vi "RPi HMI Com.vi"(0 "Pump Data":T6={"Voltages"=[0.0, 0.05908203125, 0.06982421875, 0.05908203125, 0.06982421875, 0.0859375], "PumpCurrent"=[0.0015967955457961394, 0.0015950073791676203, 0.0015981739242389562, 0.0015920643549248493, 0.001590499709124895, 0.0015808510600251774], "Speed"=[0.0, 0.0, 0.0, 0.0, 0.0, 0.0], "ControllerCurrent"=[0.0, 0.0, 0.0, 0.0, 0.0, 0.0], "Pressure"=[0.0, 0.0, 0.0, 0.0, 0.0, 0.0], "Flow"=[0.0, 0.0, 0.0, 0.0, 0.0, 0.0], "Elapsed Time (Display)"=[4074.9003000000002, 4074.9003000000002, 4074.9003000000002, 4074.9003000000002, 4074.9003000000002, 4074.9003000000002], "Avg Pressure"=0.0, "Avg Speed"=0.0, "Elapsed Time"=[4074.9003000000002, 4074.9003000000002, 4074.9003000000002, 4074.9003000000002, 4074.9003000000002, 4074.9003000000002]} {"Elapsed Time" format="%<%H:%M:%S>t"; "Elapsed Time (Display)" format="%<%H:%M:%S>t"; "Speed" format="%#_4f"; "ControllerCurrent" format="%#.1g"; "Pressure" format="%#.0f"; "Flow" format="%#.0f"; "PumpCurrent" format="%#.1g"; "Voltages" format="%#.0f"}, 1 "Tank Data":T12 {"PS Actual (V):" format="%.2f"; "Temp1" format="%#_2g"; "Temp2" format="%#_2g"}, 2 "Power Relays":T11, 3 "Pump CMDs":dbl[](array[numeric]), 4 "App Config":T1={"Location"="", "Profiles Path"=path "", "Current Profile"="", "CA Number"="", "Cycles Completed"=0, "Controller Type:"=enum."Kuhnke", "Stagger Time (ms)"=0, "Tank 1 Fuel"="", "Tank 2 Fuel"="", "Serial Numbers"={"Position 1 SN"="", "Position 2 SN"="", "Poaition 3 SN"="", "Position 4 SN"="", "Position 5 SN"="", "Position 6 SN"=""}, "Pumps Present"={"Pump 1"=FALSE, "Pump 2"=FALSE, "Pump 3"=FALSE, "Pump 4"=FALSE, "Pump 5"=FALSE, "Pump 6"=FALSE}, "VoltCtrlRef"="", "VoltageSelect"=FALSE, "Watlow Present"=FALSE, "Temp 1"=0.0, "Temp 2"=0.0, "V_Run PI?"=FALSE, "Voltage Limits"={"V_Step"=1e-05, "V_CmdMax"=0.0, "V_CmdMin"=0.0}, "Voltage Far PI"={"V_FarSlew"=10.0, "V_FarKp"=0.0, "V_FarKi"=0.0}, "Voltage Mid PI"={"V_MidSlew"=10.0, "V_MidKp"=0.0, "V_MidKi"=0.0}, "Voltage Close PI"={"V_CloseSlew"=10.0, "V_CloseKp"=0.0, "V_CloseKi"=0.0}, "Voltage Scale"={"V_FFm"=0.0, "V_FFb"=0.0}, "Voltage Cutoffs"={"V_MidCutoff"=0.0, "V_CloseCutoff"=0.0}, "Pressure Scale"={"Pres_FFm"=1e-05, "Pres_FFb"=0.0}, "Temp Format"=0, "Temp Tolerance"=0.0, "Target Voltage"=0.0, "Target Pressure"=0.0, "Data Log Init"={"Data Path"=path "", "Data Log Rate (S/s)"=0, "AKLH Rate (Hours/S)"=0.0, "Sync Time Offset (min)"=0, "IP Last 3"=0, "WebDAV IP"=""}, "Email Handler IP"="", "ADC Check"=FALSE, "3 Pump Tank"=FALSE, "Cycle Threshold:"=3.0, "Cycle Pts to Avg:"=3, "Anomaly Threshold:"=3.0, "Normal Steps:"=3, "Step Threshold:"=3.0, "Network Drive IP"="", "Network Drive Password"="", "Bank 1 Offset"=0.0, "Bank 2 Offset"=0.0} {"Bank 2 Offset" min=0.0 max=999999.0 step=1.0; "Bank 1 Offset" min=0.0 max=999999.0 step=1.0; "Step Threshold:" min=0.0 max=999999.0 step=1.0; "Normal Steps:" max=999999 step=1; "Anomaly Threshold:" min=0.0 max=999999.0 step=1.0; "Cycle Pts to Avg:" max=999999 step=1; "Cycle Threshold:" min=0.0 max=999999.0 step=1.0}, 5 "Tank CMDs":T8, 6 "Alarm":bool, 7 "HMI Tog Buttons":T9, 8 "RPi HMI Mode":T13, 9 "In Test":bool, 10 "Alarm Message 1":string, 11 "Controller Config":T4, 12 "Alarm Message 2":string, 13 "Recording":bool, 15 "Pumps Present":bool[](array[boolean]), 19 "Time/Date":string) -> (14 "HMI Cluster":T5={"Error"={"status"=FALSE, "code"=0, "source"=""}, "COM Ref"="", "Pump Data"={"Voltages"=[], "PumpCurrent"=[], "Speed"=[], "ControllerCurrent"=[], "Pressure"=[], "Flow"=[], "Elapsed Time (Display)"=[], "Avg Pressure"=0.0, "Avg Speed"=0.0, "Elapsed Time"=[4074.9003000000002, 4074.9003000000002, 4074.9003000000002, 4074.9003000000002, 4074.9003000000002, 4074.9003000000002]}, "Tank Data"={"PS Actual (V):"=0.0, "Temp1"=0.0, "Temp2"=0.0}, "Power Relays"={"Pump 1"=FALSE, "Pump 2"=FALSE, "Pump 3"=FALSE, "Pump 4"=FALSE, "Pump 5"=FALSE, "Pump 6"=FALSE}, "Pump CMDs"=[], "HMI Header"={"Line 1"="", "Line 2"="", "Line 3"="", "Line 4"=""}, "Tank CMDs"={"PS CMD"=0.0, "Press CMD"=0.0, "Temp 1 CMD"=0.0, "Temp 2 CMD"=0.0}, "HMI Tog Buttons"={"Start Test"=FALSE, "Toggle Spare 1"=FALSE, "Toggle Spare 2"=FALSE, "Toggle Spare 3"=FALSE, "Toggle Spare 4"=FALSE, "Toggle Spare 5"=FALSE}, "In Test"=FALSE, "HMI Command"=FALSE, "HMI Mom Buttons"={"Stop"=FALSE, "Reset Timers"=FALSE, "Log Fuel Change"=FALSE, "Alarm Dismiss"=FALSE}, "Controller Config"={"Controller Name"=enum."Kuhnke", "CommSeg"=0, "PWM?"=FALSE, "Frequency"=0, "Low Command"=0.0, "High Command"=0.0, "Stop Command"=0.0, "Command Step"=0.0, "Solenoid Stop?"=FALSE, "Controller?"=FALSE, "Invert PWM"=FALSE}, "Alarm"=FALSE, "Alarm Message 1"="", "Alarm Message 2"="", "Recording"=FALSE, "Serial Numbers"=[], "Pumps Present"=[]} {"Pump Data"."Elapsed Time" format="%<%H:%M:%S>t"; "Pump Data"."Elapsed Time (Display)" format="%<%H:%M:%S>t"; "Pump Data"."Speed" format="%#_4f"; "Pump Data"."ControllerCurrent" format="%#.1g"; "Pump Data"."Pressure" format="%#.0f"; "Pump Data"."Flow" format="%#.0f"; "Pump Data"."PumpCurrent" format="%#.1g"; "Pump Data"."Voltages" format="%#.0f"})   [LabVIEW 2018]
uses:
  Controls/RPi HMI Mode.ctl
  Controls/Pump Data.ctl
  Controls/Tank Data.ctl
  Controls/Tank CMDs.ctl
  Controls/HMI Tog Buttons.ctl
  Controls/HMI Cluster.ctl
  Controls/HMI Header.ctl
  Controls/HMI Mom Buttons.ctl
  Controls/Controller Config.ctl
  Type Defs/Controller Names.ctl
  Type Defs/App Config.ctl
  Data Logger/Data Log Init.ctl
  <vilib>/Instr/_visa.llb/VISA Configure Serial Port (Instr).vi
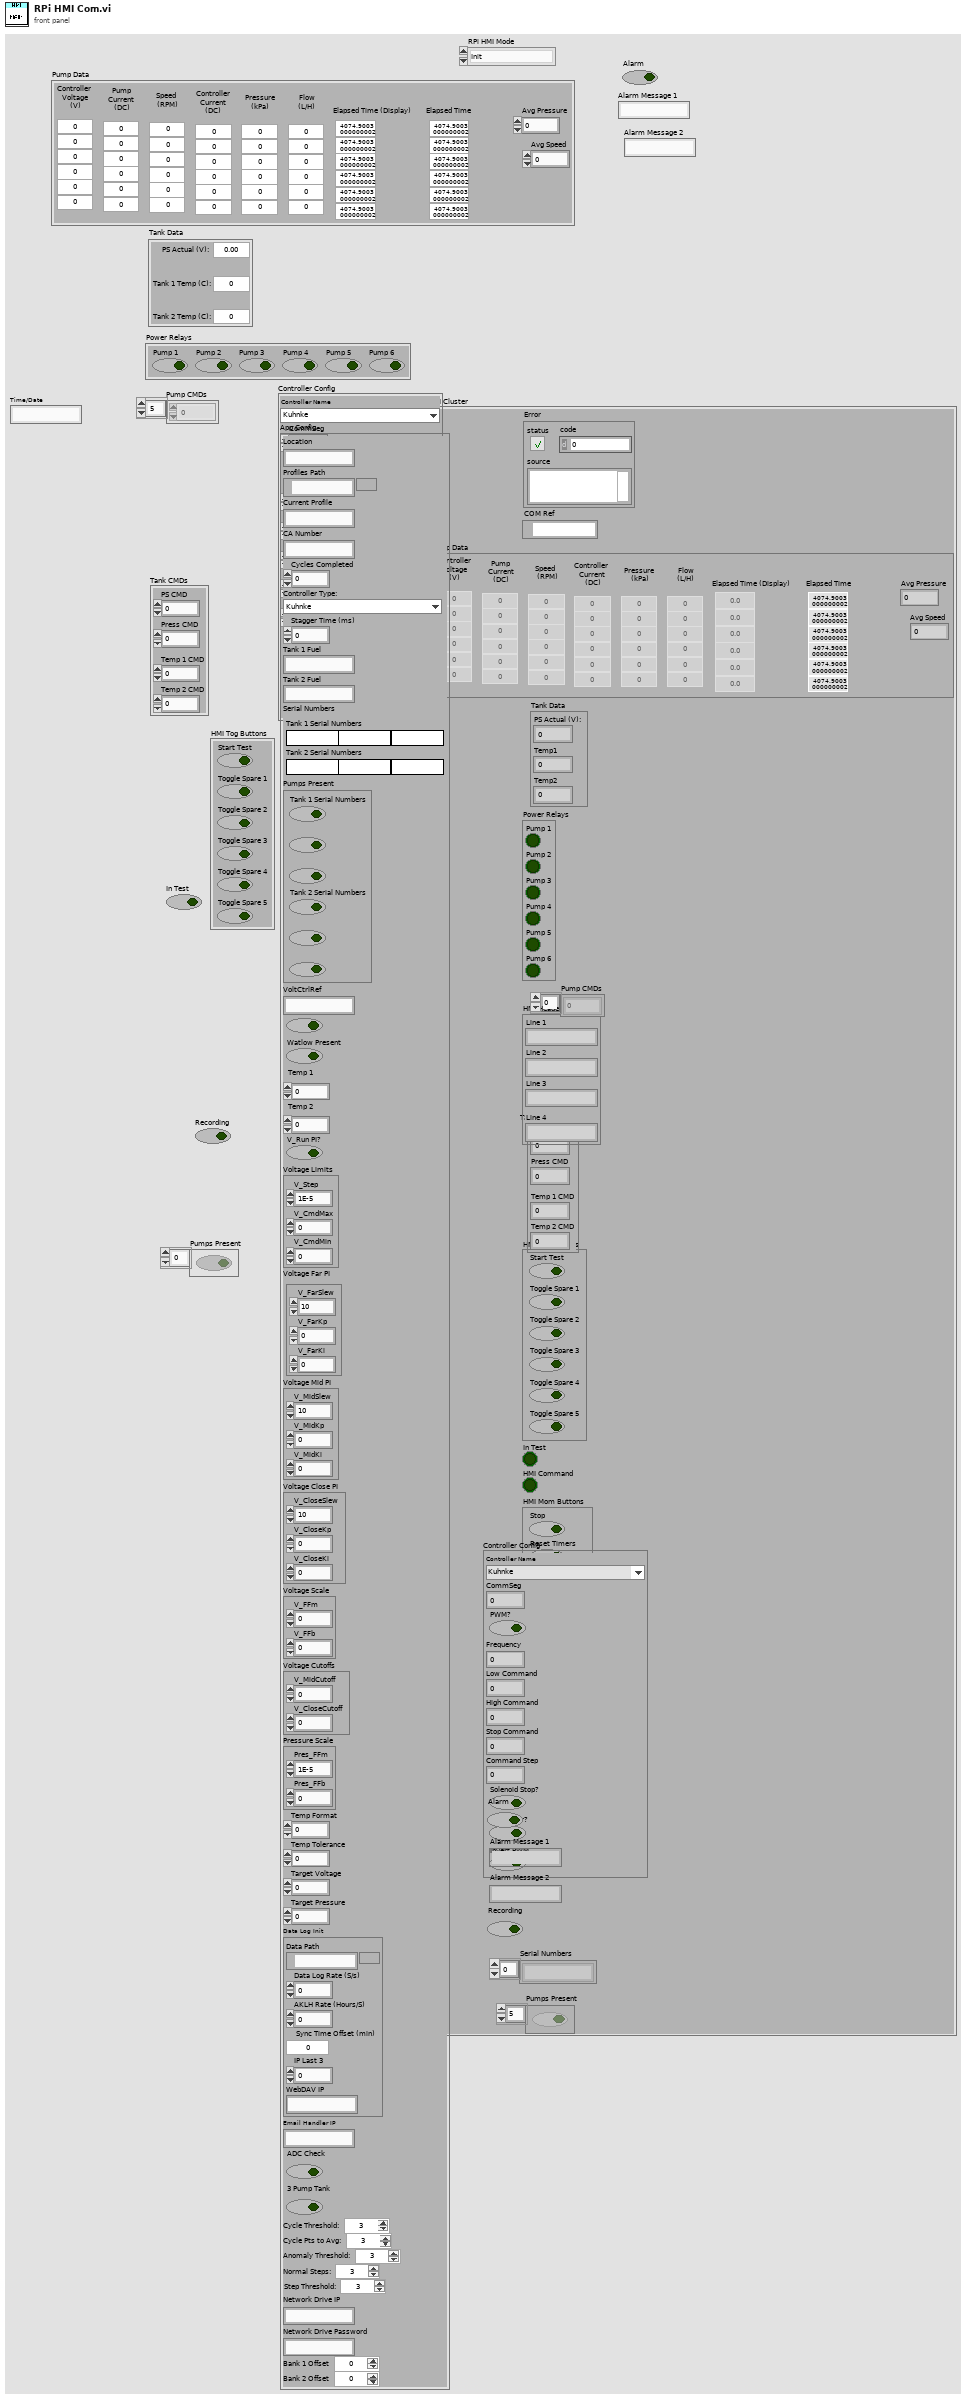
[diagram p1: front panel]
types:
  T1 = typedef "App Config.ctl" = cluster{"Location":string, "Profiles Path":path, "Current Profile":string, "CA Number":string, "Cycles Completed":u32, "Controller Type:":T2, "Stagger Time (ms)":i32, "Tank 1 Fuel":string, "Tank 2 Fuel":string, "Serial Numbers":cluster{"Position 1 SN":string, "Position 2 SN":string, "Poaition 3 SN":string, "Position 4 SN":string, "Position 5 SN":string, "Position 6 SN":string}, "Pumps Present":cluster{"Pump 1":bool, "Pump 2":bool, "Pump 3":bool, "Pump 4":bool, "Pump 5":bool, "Pump 6":bool}, "VoltCtrlRef":string, "VoltageSelect":bool, "Watlow Present":bool, "Temp 1":dbl, "Temp 2":dbl, "V_Run PI?":bool, "Voltage Limits":cluster{"V_Step":dbl, "V_CmdMax":dbl, "V_CmdMin":dbl}, "Voltage Far PI":cluster{"V_FarSlew":dbl, "V_FarKp":dbl, "V_FarKi":dbl}, "Voltage Mid PI":cluster{"V_MidSlew":dbl, "V_MidKp":dbl, "V_MidKi":dbl}, "Voltage Close PI":cluster{"V_CloseSlew":dbl, "V_CloseKp":dbl, "V_CloseKi":dbl}, "Voltage Scale":cluster{"V_FFm":dbl, "V_FFb":dbl}, "Voltage Cutoffs":cluster{"V_MidCutoff":dbl, "V_CloseCutoff":dbl}, "Pressure Scale":cluster{"Pres_FFm":dbl, "Pres_FFb":dbl}, "Temp Format":i32, "Temp Tolerance":dbl, "Target Voltage":dbl, "Target Pressure":dbl, "Data Log Init":T3, "Email Handler IP":string, "ADC Check":bool, "3 Pump Tank":bool, "Cycle Threshold:":dbl, "Cycle Pts to Avg:":i32, "Anomaly Threshold:":dbl, "Normal Steps:":u32, "Step Threshold:":dbl, "Network Drive IP":string, "Network Drive Password":string, "Bank 1 Offset":dbl, "Bank 2 Offset":dbl}
  T2 = typedef "Controller Names.ctl" = enum16{"Kuhnke", "Helbako BLDC", "Conti", "Hella BLDC OL PWM", "Hella BLDC Turbine OL PWM", "Hella BLDC Pressure", "Helbako (old)", "TI PWM", "PSA", "Hella Gas", "Hella Diesel", "8 Comm", "10 Comm", "8 Comm Hella", "10 Comm Hella", "8 Comm Omron", "10 Comm Omron", "8 Comm Nissan", "10 Comm Nissan"}
  T3 = typedef "Data Log Init.ctl" = cluster{"Data Path":path, "Data Log Rate (S/s)":u32, "AKLH Rate (Hours/S)":dbl, "Sync Time Offset (min)":i32, "IP Last 3":i32, "WebDAV IP":string}
  T4 = typedef "Controller Config.ctl" = cluster{"Controller Name":T2, "CommSeg":i32, "PWM?":bool, "Frequency":i32, "Low Command":dbl, "High Command":dbl, "Stop Command":dbl, "Command Step":dbl, "Solenoid Stop?":bool, "Controller?":bool, "Invert PWM":bool}
  T5 = typedef "HMI Cluster.ctl" = cluster{"Error":errorcluster, "COM Ref":refnum<visa-resource-name>, "Pump Data":T6, "Tank Data":cluster{"PS Actual (V):":dbl, "Temp1":dbl, "Temp2":dbl}, "Power Relays":cluster{"Pump 1":bool, "Pump 2":bool, "Pump 3":bool, "Pump 4":bool, "Pump 5":bool, "Pump 6":bool}, "Pump CMDs":dbl[], "HMI Header":T7, "Tank CMDs":T8, "HMI Tog Buttons":T9, "In Test":bool, "HMI Command":bool, "HMI Mom Buttons":T10, "Controller Config":T4, "Alarm":bool, "Alarm Message 1":string, "Alarm Message 2":string, "Recording":bool, "Serial Numbers":string[], "Pumps Present":bool[]}
  T6 = typedef "Pump Data.ctl" = cluster{"Voltages":dbl[], "PumpCurrent":dbl[], "Speed":dbl[], "ControllerCurrent":dbl[], "Pressure":dbl[], "Flow":dbl[], "Elapsed Time (Display)":dbl[], "Avg Pressure":dbl, "Avg Speed":dbl, "Elapsed Time":dbl[]}
  T7 = typedef "HMI Header.ctl" = cluster{"Line 1":string, "Line 2":string, "Line 3":string, "Line 4":string}
  T8 = typedef "Tank CMDs.ctl" = cluster{"PS CMD":dbl, "Press CMD":dbl, "Temp 1 CMD":dbl, "Temp 2 CMD":dbl}
  T9 = typedef "HMI Tog Buttons.ctl" = cluster{"Start Test":bool, "Toggle Spare 1":bool, "Toggle Spare 2":bool, "Toggle Spare 3":bool, "Toggle Spare 4":bool, "Toggle Spare 5":bool}
  T10 = typedef "HMI Mom Buttons.ctl" = cluster{"Stop":bool, "Reset Timers":bool, "Log Fuel Change":bool, "Alarm Dismiss":bool}
  T11 = cluster{"Pump 1":bool, "Pump 2":bool, "Pump 3":bool, "Pump 4":bool, "Pump 5":bool, "Pump 6":bool}
  T12 = typedef "Tank Data.ctl" = cluster{"PS Actual (V):":dbl, "Temp1":dbl, "Temp2":dbl}
  T13 = typedef "RPi HMI Mode.ctl" = enum16{"Init", "Write Data", "Read from RPi", "Write to RPi"}
  T14 = cluster{"PS Actual (V):":dbl, "Temp1":dbl, "Temp2":dbl}
  T15 = cluster{"Position 1 SN":string, "Position 2 SN":string, "Poaition 3 SN":string, "Position 4 SN":string, "Position 5 SN":string, "Position 6 SN":string}
  T16 = cluster{"Tank CMDs[0]":dbl, "Tank CMDs[1]":dbl, "Tank CMDs[2]":dbl, "Tank CMDs[3]":dbl}
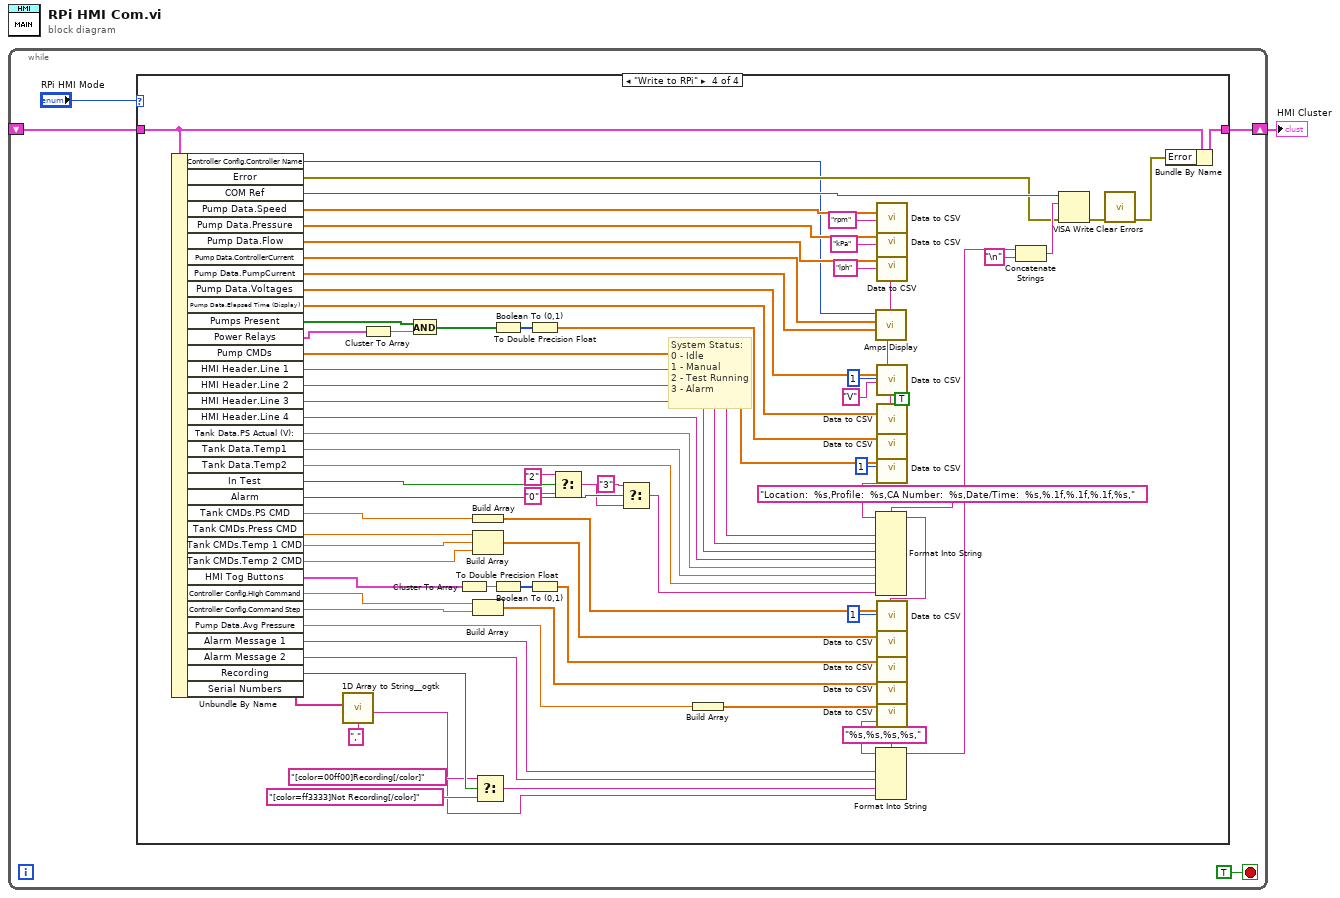
[diagram p0: block diagram]
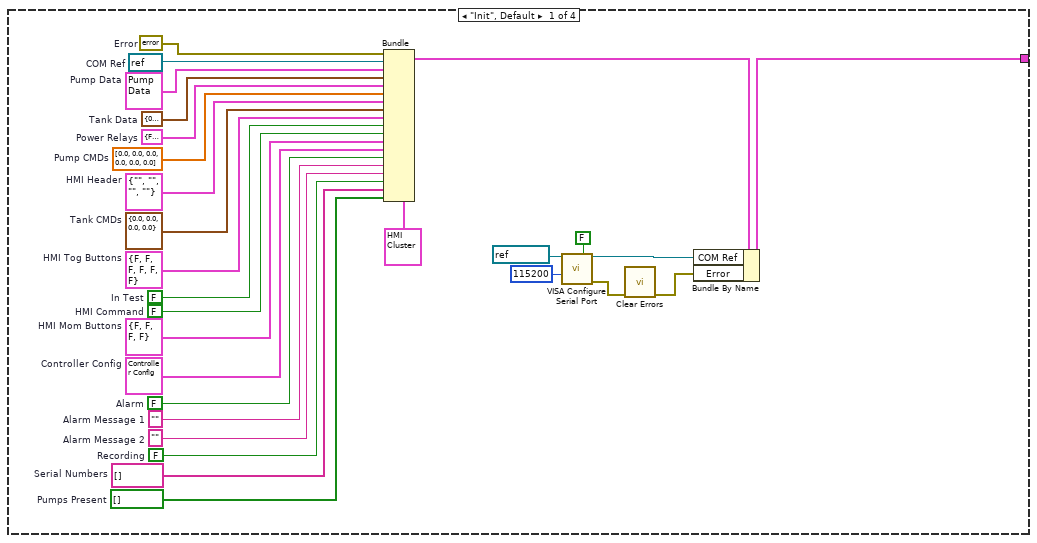
[diagram p2: hidden frame]
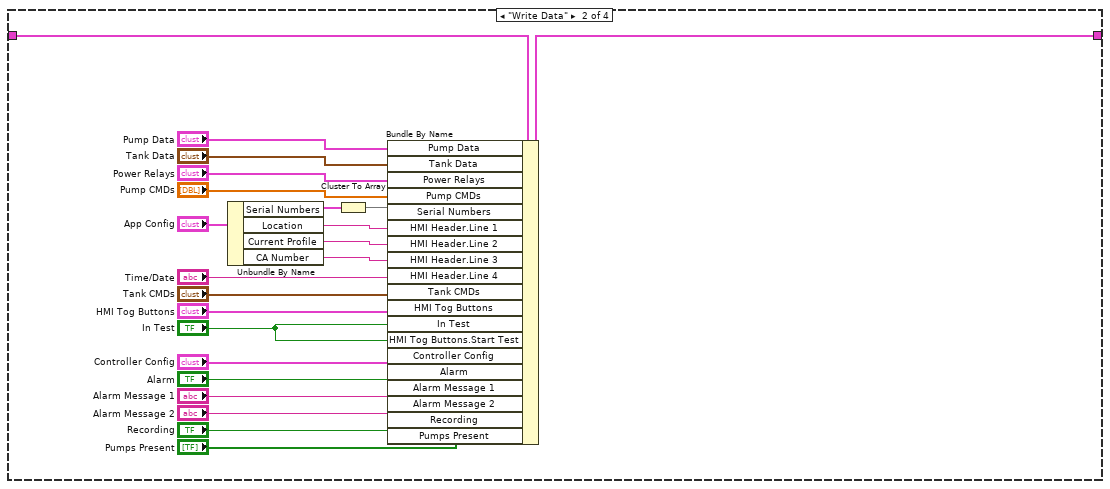
[diagram p3: hidden frame]
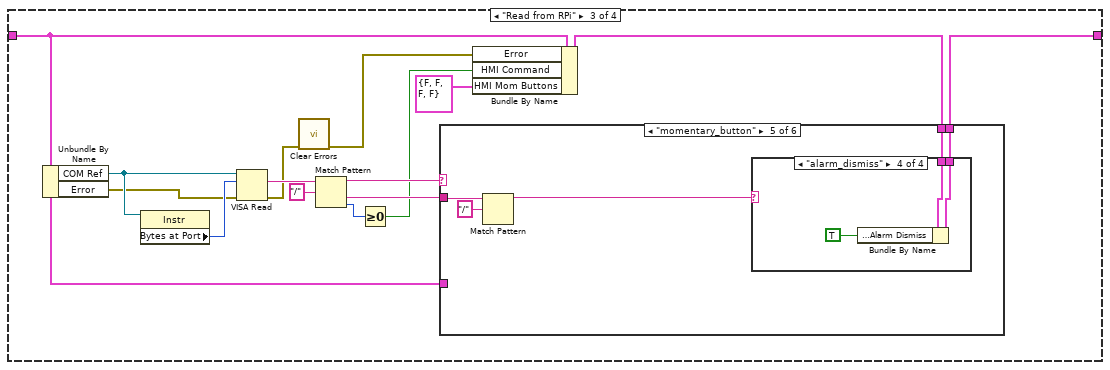
[diagram p4: hidden frame]
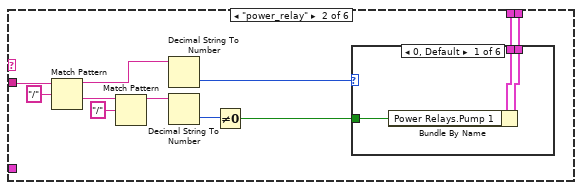
[diagram p6: hidden frame]
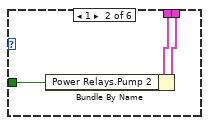
[diagram p7: hidden frame]
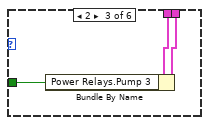
[diagram p8: hidden frame]
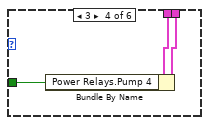
[diagram p9: hidden frame]
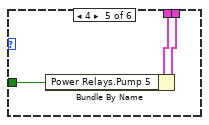
[diagram p10: hidden frame]
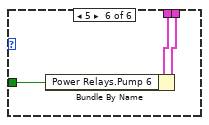
[diagram p11: hidden frame]
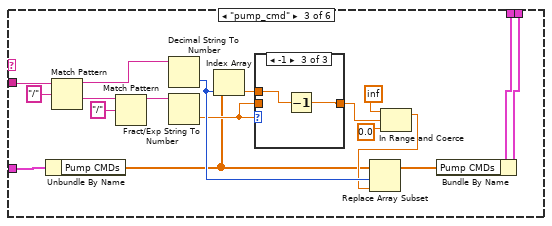
[diagram p12: hidden frame]
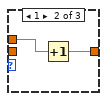
[diagram p14: hidden frame]
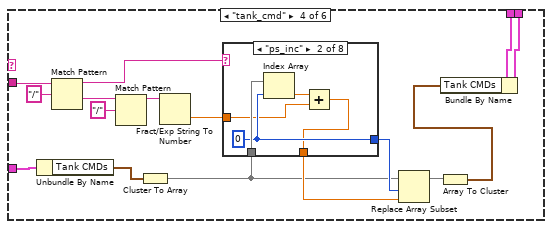
[diagram p15: hidden frame]
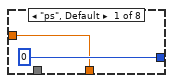
[diagram p16: hidden frame]
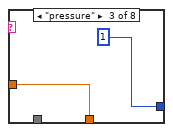
[diagram p17: hidden frame]
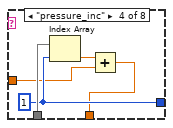
[diagram p18: hidden frame]
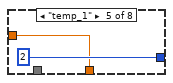
[diagram p19: hidden frame]
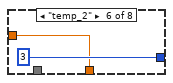
[diagram p20: hidden frame]
diagram:
  n1 = while {
    shift-right: [w3] -> w1
    shift-left: _ -> [w2]
    stop <- TRUE stop-if-true
    n2 = case shown="\"Write to RPi\"" "RPi HMI Mode" {
      tunnel: [w27 w54 w62 w242] -> w3
      tunnel: w2 -> [_ w55 w60 w243]
      frame "Init", Default {
        w6 = T4 {"Controller Name"=enum."Kuhnke", "CommSeg"=0, "PWM?"=FALSE, "Frequency"=0, "Low Command"=0.0, "High Command"=0.0, "Stop Command"=0.0, "Command Step"=0.0, "Solenoid Stop?"=FALSE, "Controller?"=FALSE, "Invert PWM"=FALSE}  # Controller Config
        w7 = bool[] []  # Pumps Present
        w8 = string[] []  # Serial Numbers
        w9 = FALSE  # Recording
        w10 = ""  # Alarm Message 2
        w11 = ""  # Alarm Message 1
        w12 = FALSE  # Alarm
        w16 = T10 {"Stop"=FALSE, "Reset Timers"=FALSE, "Log Fuel Change"=FALSE, "Alarm Dismiss"=FALSE}  # HMI Mom Buttons
        w17 = T11 {"Pump 1"=FALSE, "Pump 2"=FALSE, "Pump 3"=FALSE, "Pump 4"=FALSE, "Pump 5"=FALSE, "Pump 6"=FALSE}  # Power Relays
        w18 = FALSE  # HMI Command
        w19 = FALSE  # In Test
        w20 = T9 {"Start Test"=FALSE, "Toggle Spare 1"=FALSE, "Toggle Spare 2"=FALSE, "Toggle Spare 3"=FALSE, "Toggle Spare 4"=FALSE, "Toggle Spare 5"=FALSE}  # HMI Tog Buttons
        w21 = T8 {"PS CMD"=0.0, "Press CMD"=0.0, "Temp 1 CMD"=0.0, "Temp 2 CMD"=0.0}  # Tank CMDs
        w22 = T7 {"Line 1"="", "Line 2"="", "Line 3"="", "Line 4"=""}  # HMI Header
        w23 = T14 {"PS Actual (V):"=0.0, "Temp1"=0.0, "Temp2"=0.0}  # Tank Data
        w24 = dbl[] [0.0, 0.0, 0.0, 0.0, 0.0, 0.0]  # Pump CMDs
        w25 = errorcluster {"status"=FALSE, "code"=0, "source"=""}  # Error
        w29 = T6 {"Voltages"=[0.0, 0.05908203125, 0.06982421875, 0.05908203125, 0.06982421875, 0.0859375], "PumpCurrent"=[0.0015967955457961394, 0.0015950073791676203, 0.0015981739242389562, 0.0015920643549248493, 0.001590499709124895, 0.0015808510600251774], "Speed"=[0.0, 0.0, 0.0, 0.0, 0.0, 0.0], "ControllerCurrent"=[0.0, 0.0, 0.0, 0.0, 0.0, 0.0], "Pressure"=[0.0, 0.0, 0.0, 0.0, 0.0, 0.0], "Flow"=[0.0, 0.0, 0.0, 0.0, 0.0, 0.0], "Elapsed Time (Display)"=[4074.9003000000002, 4074.9003000000002, 4074.9003000000002, 4074.9003000000002, 4074.9003000000002, 4074.9003000000002], "Avg Pressure"=0.0, "Avg Speed"=0.0, "Elapsed Time"=[]}  # Pump Data
        w30 = refnum<visa-resource-name> refnum  # COM Ref
        n3 = Bundle(cluster=T5 {"Error"={"status"=FALSE, "code"=0, "source"=""}, "COM Ref"="", "Pump Data"={"Voltages"=[], "PumpCurrent"=[], "Speed"=[], "ControllerCurrent"=[], "Pressure"=[], "Flow"=[], "Elapsed Time (Display)"=[], "Avg Pressure"=0.0, "Avg Speed"=0.0, "Elapsed Time"=[]}, "Tank Data"={"PS Actual (V):"=0.0, "Temp1"=0.0, "Temp2"=0.0}, "Power Relays"={"Pump 1"=FALSE, "Pump 2"=FALSE, "Pump 3"=FALSE, "Pump 4"=FALSE, "Pump 5"=FALSE, "Pump 6"=FALSE}, "Pump CMDs"=[], "HMI Header"={"Line 1"="", "Line 2"="", "Line 3"="", "Line 4"=""}, "Tank CMDs"={"PS CMD"=0.0, "Press CMD"=0.0, "Temp 1 CMD"=0.0, "Temp 2 CMD"=0.0}, "HMI Tog Buttons"={"Start Test"=FALSE, "Toggle Spare 1"=FALSE, "Toggle Spare 2"=FALSE, "Toggle Spare 3"=FALSE, "Toggle Spare 4"=FALSE, "Toggle Spare 5"=FALSE}, "In Test"=FALSE, "HMI Command"=FALSE, "HMI Mom Buttons"={"Stop"=FALSE, "Reset Timers"=FALSE, "Log Fuel Change"=FALSE, "Alarm Dismiss"=FALSE}, "Controller Config"={"Controller Name"=enum."Kuhnke", "CommSeg"=0, "PWM?"=FALSE, "Frequency"=0, "Low Command"=0.0, "High Command"=0.0, "Stop Command"=0.0, "Command Step"=0.0, "Solenoid Stop?"=FALSE, "Controller?"=FALSE, "Invert PWM"=FALSE}, "Alarm"=FALSE, "Alarm Message 1"="", "Alarm Message 2"="", "Recording"=FALSE, "Serial Numbers"=[], "Pumps Present"=[]} ("HMI Cluster"), "Error"=w25, "COM Ref"=w30, "Pump Data"=w29, "Tank Data"=w23, "Power Relays"=w17, "Pump CMDs"=w24, "HMI Header"=w22, "Tank CMDs"=w21, "HMI Tog Buttons"=w20, "In Test"=w19, "HMI Command"=w18, "HMI Mom Buttons"=w16, "Controller Config"=w6, "Alarm"=w12, "Alarm Message 1"=w11, "Alarm Message 2"=w10, "Recording"=w9, "Serial Numbers"=w8, "Pumps Present"=w7) -> (w28:T5)
        n4 = call-poly "VISA Configure Serial Port"("VISA resource name"=refnum<visa-resource-name> "COM1", "Enable Termination\nChar (T)"=FALSE ("Enable Termination\nChar (T)"), "baud rate (9600)"=u32 115200) -> ("VISA resource name out"=w26:refnum<visa-resource-name>, "error out"=w14:errorcluster)  [unwired: 11 in]
        n5 = call <vilib>:"Clear Errors.vi"("error in (no error)"=w14) -> ("error out"=w13:errorcluster)  [unwired: 5 in, 1 out]
        n6 = Bundle By Name(cluster=w28, "COM Ref"=w26, "Error"=w13) -> (w27:T5)
      }
      frame "Write Data" {
        n7 = Unbundle By Name("App Config") -> ("Serial Numbers"=w35:T15, "Location"=w39:string, "Current Profile"=w38:string, "CA Number"=w37:string)
        n8 = Cluster To Array(cluster=w35) -> (array=w34:string[])
        n9 = Bundle By Name(cluster=w55, "Pump Data"="Pump Data", "Tank Data"="Tank Data", "Power Relays"="Power Relays", "Pump CMDs"="Pump CMDs", "Serial Numbers"=w34, "HMI Header.Line 1"=w39, "HMI Header.Line 2"=w38, "HMI Header.Line 3"=w37, "HMI Header.Line 4"="Time/Date", "Tank CMDs"="Tank CMDs", "HMI Tog Buttons"="HMI Tog Buttons", "In Test"="In Test", "HMI Tog Buttons.Start Test"="In Test", "Controller Config"="Controller Config", "Alarm"="Alarm", "Alarm Message 1"="Alarm Message 1", "Alarm Message 2"="Alarm Message 2", "Recording"="Recording", "Pumps Present"="Pumps Present") -> (w54:T5)
      }
      frame "Read from RPi" {
        n10 = Unbundle By Name(w60) -> ("COM Ref"=w67:refnum<visa-resource-name>, "Error"=w58:errorcluster)
        n11 = property class="Instr"(reference=w67) -> ("Bytes at Port"=w68:u32)  [unwired: 1 in, 2 out]
        n12 = VISA Read(VISA resource name=w67, byte count=w68, error in (no error)=w58) -> (read buffer=w69:string, error out=w57:errorcluster)  [unwired: 2 out]
        n13 = call <vilib>:"Clear Errors.vi"("error in (no error)"=w57) -> ("error out"=w56:errorcluster)  [unwired: 5 in, 1 out]
        n14 = Match Pattern(string=w69, regular expression="/") -> (before substring=w66:string, after substring=w65:string, offset past match=w64:i32)  [unwired: 1 in, 1 out]
        n15 = Greater Or Equal To 0?(x=w64) -> (x >= 0?=w63:bool)
        n16 = Bundle By Name(cluster=w60, "Error"=w56, "HMI Command"=w63, "HMI Mom Buttons"=T10 {"Stop"=FALSE, "Reset Timers"=FALSE, "Log Fuel Change"=FALSE, "Alarm Dismiss"=FALSE}) -> (w61:T5)
        n17 = case shown="\"momentary_button\"" w66 {
          tunnel: w65 -> [_ w81 w117 w138 w171 w193]
          tunnel: w61 -> [w71 w75 w104 w126 w169 w191]
          tunnel: [w71 w74 w103 w125 w168 w190] -> w62
          tunnel: w60 -> [_ _ w101 w130 _ _]
          frame "null", Default {
          }
          frame "power_relay" {
            n18 = Match Pattern(string=w81, regular expression="/") -> (before substring=w76:string, after substring=w79:string)  [unwired: 1 in, 2 out]
            n19 = Match Pattern(string=w79, regular expression="/") -> (before substring=w78:string)  [unwired: 1 in, 3 out]
            n20 = Decimal String To Number(string=w76) -> (number=w73:i32)  [unwired: 2 in, 1 out]
            n21 = Decimal String To Number(string=w78) -> (number=w77:i32)  [unwired: 2 in, 1 out]
            n22 = Not Equal To 0?(x=w77) -> (x != 0?=w72:bool)
            n23 = case shown="0, Default" w73 {
              tunnel: w75 -> [w85 w88 w91 w94 w97 w100]
              tunnel: [w84 w87 w90 w93 w96 w99] -> w74
              tunnel: w72 -> [w83 w86 w89 w92 w95 w98]
              frame 0, Default {
                n24 = Bundle By Name(cluster=w85, "Power Relays.Pump 1"=w83) -> (w84:T5)
              }
              frame 1 {
                n25 = Bundle By Name(cluster=w88, "Power Relays.Pump 2"=w86) -> (w87:T5)
              }
              frame 2 {
                n26 = Bundle By Name(cluster=w91, "Power Relays.Pump 3"=w89) -> (w90:T5)
              }
              frame 3 {
                n27 = Bundle By Name(cluster=w94, "Power Relays.Pump 4"=w92) -> (w93:T5)
              }
              frame 4 {
                n28 = Bundle By Name(cluster=w97, "Power Relays.Pump 5"=w95) -> (w96:T5)
              }
              frame 5 {
                n29 = Bundle By Name(cluster=w100, "Power Relays.Pump 6"=w98) -> (w99:T5)
              }
            }
          }
          frame "pump_cmd" {
            n30 = Unbundle By Name(w101) -> ("Pump CMDs"=w105:dbl[])
            n31 = Match Pattern(string=w117, regular expression="/") -> (before substring=w113:string, after substring=w115:string)  [unwired: 1 in, 2 out]
            n32 = Match Pattern(string=w115, regular expression="/") -> (before substring=w114:string)  [unwired: 1 in, 3 out]
            n33 = Decimal String To Number(string=w113) -> (number=w111:i32)  [unwired: 2 in, 1 out]
            n34 = Fract/Exp String To Number(string=w114) -> (number=w110:dbl)  [unwired: 3 in, 1 out]
            n35 = Index Array(array=w105, index=w111) -> (element=w112:dbl)
            n36 = case shown="-1" w110 {
              tunnel: w112 -> [_ w121 w123]
              tunnel: w110 -> [w119 _ _]
              tunnel: [w119 w120 w122] -> w109
              frame 0, Default {
              }
              frame 1 {
                n37 = Increment(x=w121) -> (x+1=w120:dbl)
              }
              frame -1 {
                n38 = Decrement(x=w123) -> (x-1=w122:dbl)
              }
            }
            n39 = In Range and Coerce(upper limit=inf, x=w109, lower limit=0.0) -> (coerced(x)=w106:dbl)  [unwired: 1 out]
            n40 = Replace Array Subset(array=w105, new element=w106, index=w111) -> (w102:dbl[])
            n41 = Bundle By Name(cluster=w104, "Pump CMDs"=w102) -> (w103:T5)
          }
          frame "tank_cmd" {
            n42 = Unbundle By Name(w130) -> ("Tank CMDs"=w129:T8)
            n43 = Match Pattern(string=w138, regular expression="/") -> (before substring=w134:string, after substring=w136:string)  [unwired: 1 in, 2 out]
            n44 = Match Pattern(string=w136, regular expression="/") -> (before substring=w135:string)  [unwired: 1 in, 3 out]
            n45 = Cluster To Array(cluster=w129) -> (array=w128:dbl[])
            n46 = Fract/Exp String To Number(string=w135) -> (number=w131:dbl)  [unwired: 3 in, 1 out]
            n47 = case shown="\"ps_inc\"" w134 {
              tunnel: [0 w145 1 w152 2 3 w161 w166] -> w133
              tunnel: [w140 w142 w147 w149 w154 w156 w158 w163] -> w132
              tunnel: w131 -> [w140 w143 w147 w150 w154 w156 w159 w164]
              tunnel: w128 -> [_ w146 _ w153 _ _ w162 w167]
              frame "ps", Default {
              }
              frame "ps_inc" {
                w145 = 0
                n48 = Index Array(array=w146, index=w145) -> (element=w144:dbl)
                n49 = Add(x=w144, y=w143) -> (x+y=w142:dbl)
              }
              frame "pressure" {
              }
              frame "pressure_inc" {
                w152 = 1
                n50 = Index Array(array=w153, index=w152) -> (element=w151:dbl)
                n51 = Add(x=w151, y=w150) -> (x+y=w149:dbl)
              }
              frame "temp_1" {
              }
              frame "temp_2" {
              }
              frame "temp_1_inc" {
                w161 = 2
                n52 = Index Array(array=w162, index=w161) -> (element=w160:dbl)
                n53 = Add(x=w160, y=w159) -> (x+y=w158:dbl)
              }
              frame "temp_2_inc" {
                w166 = 3
                n54 = Index Array(array=w167, index=w166) -> (element=w165:dbl)
                n55 = Add(x=w165, y=w164) -> (x+y=w163:dbl)
              }
            }
            n56 = Replace Array Subset(array=w128, new element=w132, index=w133) -> (w127:dbl[])
            n57 = Array To Cluster(array=w127) -> (cluster=w124:T16)
            n58 = Bundle By Name(cluster=w126, "Tank CMDs"=w124) -> (w125:T5)
          }
          frame "momentary_button" {
            n59 = Match Pattern(string=w171, regular expression="/") -> (before substring=w170:string)  [unwired: 1 in, 3 out]
            n60 = case shown="\"alarm_dismiss\"" w170 {
              tunnel: w169 -> [w175 w177 w180 w183]
              tunnel: [w174 w176 w179 w182] -> w168
              frame "stop", Default {
                n61 = Bundle By Name(cluster=w175, "HMI Mom Buttons.Stop"=TRUE) -> (w174:T5)
              }
              frame "reset_timers" {
                n62 = Bundle By Name(cluster=w177, "HMI Mom Buttons.Reset Timers"=TRUE ("HMI Mom Buttons.Stop")) -> (w176:T5)
              }
              frame "log_fuel_change" {
                n63 = Bundle By Name(cluster=w180, "HMI Mom Buttons.Log Fuel Change"=TRUE ("HMI Mom Buttons.Stop")) -> (w179:T5)
              }
              frame "alarm_dismiss" {
                n64 = Bundle By Name(cluster=w183, "HMI Mom Buttons.Alarm Dismiss"=TRUE ("HMI Mom Buttons.Stop")) -> (w182:T5)
              }
            }
          }
          frame "toggle_button" {
            n65 = Match Pattern(string=w193, regular expression="/") -> (before substring=w192:string, after substring=w188:string)  [unwired: 1 in, 2 out]
            n66 = Match Pattern(string=w188, regular expression="/") -> (before substring=w186:string)  [unwired: 1 in, 3 out]
            n67 = Decimal String To Number(string=w186) -> (number=w187:i32)  [unwired: 2 in, 1 out]
            n68 = Not Equal To 0?(x=w187) -> (x != 0?=w185:bool)
            n69 = case shown="\"start_test\", Default" w192 {
              tunnel: w191 -> [w198 w200 w203]
              tunnel: [w197 w199 w202] -> w190
              tunnel: w185 -> [w196 _ _]
              frame "start_test", Default {
                n70 = Not(x=w196) -> (.not. x?=w195:bool)
                n71 = Bundle By Name(cluster=w198, "HMI Tog Buttons.Start Test"=w196, "HMI Mom Buttons.Stop"=w195) -> (w197:T5)
              }
              frame "reset_timers" {
                n72 = Bundle By Name(cluster=w200, "HMI Mom Buttons.Reset Timers"=TRUE ("HMI Mom Buttons.Stop")) -> (w199:T5)
              }
              frame "log_fuel_change" {
                n73 = Bundle By Name(cluster=w203, "HMI Mom Buttons.Log Fuel Change"=TRUE ("HMI Mom Buttons.Stop")) -> (w202:T5)
              }
            }
          }
        }
      }
      frame "Write to RPi" {
        # "System Status:\n0 - Idle\n1 - Manual\n2 - Test Running\n3 - Alarm"
        n74 = Unbundle By Name(w243) -> ("Controller Config.Controller Name"=w234:T2, "Error"=w244:errorcluster, "COM Ref"=w288:refnum<visa-resource-name>, "Pump Data.Speed"=w287:dbl[], "Pump Data.Pressure"=w279:dbl[], "Pump Data.Flow"=w278:dbl[], "Pump Data.ControllerCurrent"=w277:dbl[], "Pump Data.PumpCurrent"=w276:dbl[], "Pump Data.Voltages"=w275:dbl[], "Pump Data.Elapsed Time (Display)"=w272:dbl[], "Pumps Present"=w207:bool[], "Power Relays"=w246:T11, "Pump CMDs"=w270:dbl[], "HMI Header.Line 1"=w266:string, "HMI Header.Line 2"=w265:string, "HMI Header.Line 3"=w264:string, "HMI Header.Line 4"=w217:string, "Tank Data.PS Actual (V):"=w218:dbl, "Tank Data.Temp1"=w219:dbl, "Tank Data.Temp2"=w220:dbl, "In Test"=w263:bool, "Alarm"=w228:bool, "Tank CMDs.PS CMD"=w258:dbl, "Tank CMDs.Press CMD"=w257:dbl, "Tank CMDs.Temp 1 CMD"=w256:dbl, "Tank CMDs.Temp 2 CMD"=w233:dbl, "HMI Tog Buttons"=w252:T9, "Controller Config.High Command"=w239:dbl, "Controller Config.Command Step"=w238:dbl, "Pump Data.Avg Pressure"=w231:dbl, "Alarm Message 1"=w223:string, "Alarm Message 2"=w222:string, "Recording"=w216:bool, "Serial Numbers"=w211:string[])
        n75 = call <userlib>:"1D Array to String__ogtk.vi"("delimiter (Tab)"=",", "Array of Strings"=w211) -> ("delimited string"=w209:string)  [unwired: 9 in]
        n76 = Cluster To Array(cluster=w246) -> (array=w208:bool[])
        n77 = And(x=w207, y=w208) -> (x .and. y?=w206:bool[])
        n78 = Cluster To Array(cluster=w252) -> (array=w251:bool[])
        n79 = Build Array(w258) -> (w255:dbl[])
        n80 = Build Array(w257, w256, w233) -> (w253:dbl[])
        n81 = Build Array(w239, w238) -> (w205:dbl[])
        n82 = Select(t="[color=00ff00]Recording[/color]" ("Units"), s=w216, f="[color=ff3333]Not Recording[/color]" ("Units")) -> (s? t:f=w213:string)
        n83 = Boolean To (0,1)(Boolean=w206) -> (0, 1=w247:i16[])
        n84 = Boolean To (0,1)(Boolean=w251) -> (0, 1=w250:i16[])
        n85 = To Double Precision Float(number=w247) -> (double precision float=w245:dbl[])
        n86 = To Double Precision Float(number=w250) -> (double precision float=w249:dbl[])
        n87 = Select(t="2" ("Units"), s=w263, f="0" ("Units")) -> (s? t:f=w227:string)
        n88 = Select(t="3", s=w228, f=w227) -> (s? t:f=w221:string)
        n89 = Build Array(w231) -> (w230:dbl[])
        n90 = call "Data to CSV.vi"("Data Array"=w287, "Units"="rpm") -> ("String OUT"=w281:string)  [unwired: 25 in]
        n91 = call "Data to CSV.vi"("Data Array"=w279, "Units"="kPa", "String IN"=w281) -> ("String OUT"=w280:string)  [unwired: 24 in]
        n92 = call "Data to CSV.vi"("Data Array"=w278, "Units"="lph", "String IN"=w280) -> ("String OUT"=w236:string)  [unwired: 24 in]
        n93 = call "Amps Display.vi"("String IN"=w236, "Pump Current"=w276, "Controller Current"=w277, "Controller Type:"=w234) -> ("String OUT"=w235:string)  [unwired: 7 in]
        n94 = call "Data to CSV.vi"("Data Array"=w275, "Precision (0)"=i16 1, "Units"="V", "String IN"=w235) -> ("String OUT"=w273:string)  [unwired: 23 in]
        n95 = call "Data to CSV.vi"("Data Array"=w272, "String IN"=w273, "Time? (F)"=TRUE) -> ("String OUT"=w271:string)  [unwired: 24 in]
        n96 = call "Data to CSV.vi"("Data Array"=w245, "String IN"=w271) -> ("String OUT"=w269:string)  [unwired: 25 in]
        n97 = call "Data to CSV.vi"("Data Array"=w270, "Precision (0)"=i16 1, "String IN"=w269) -> ("String OUT"=w268:string)  [unwired: 24 in]
        n98 = Format Into String(format string="Location:  %s,Profile:  %s,CA Number:  %s,Date/Time:  %s,%.1f,%.1f,%.1f,%s,", initial string=w268, w266, w265, w264, w217, w218, w219, w220, w221) -> (resulting string=w259:string)  [unwired: 1 in, 1 out]
        n99 = call "Data to CSV.vi"("Data Array"=w255, "Precision (0)"=i16 1, "String IN"=w259) -> ("String OUT"=w254:string)  [unwired: 24 in]
        n100 = call "Data to CSV.vi"("Data Array"=w253, "String IN"=w254) -> ("String OUT"=w248:string)  [unwired: 25 in]
        n101 = call "Data to CSV.vi"("Data Array"=w249, "String IN"=w248) -> ("String OUT"=w237:string)  [unwired: 25 in]
        n102 = call "Data to CSV.vi"("Data Array"=w205, "String IN"=w237) -> ("String OUT"=w232:string)  [unwired: 25 in]
        n103 = call "Data to CSV.vi"("Data Array"=w230, "String IN"=w232) -> ("String OUT"=w225:string)  [unwired: 25 in]
        n104 = Format Into String(format string="%s,%s,%s,%s,", initial string=w225, w223, w222, w213, w209) -> (resulting string=w212:string)  [unwired: 1 in, 1 out]
        n105 = Concatenate Strings(w212, "\n" ("string")) -> (w290:string)
        n106 = VISA Write(VISA resource name=w288, write buffer=w290, error in (no error)=w244) -> (error out=w241:errorcluster)  [unwired: 2 out]
        n107 = call <vilib>:"Clear Errors.vi"("error in (no error)"=w241) -> ("error out"=w240:errorcluster)  [unwired: 5 in, 1 out]
        n108 = Bundle By Name(cluster=w243, "Error"=w240) -> (w242:T5)
      }
    }
  }
  "HMI Cluster" <- w1
